vi "Write X.vi"(8 "error in (no error)":errorcluster, 10 "X":variant, 11 "AssertEqualValue in":refnum<class "AssertEqualValue.lvclass">) -> (0 "error out":errorcluster, 3 "AssertEqualValue out":refnum<class "AssertEqualValue.lvclass">)   [LabVIEW 2021, in "Bananas.lvlib" / "AssertEqualValue.lvclass"]
uses:
  AssertEqualValue.lvclass
  AssertEqualValue.lvclass/AssertEqualValue.ctl
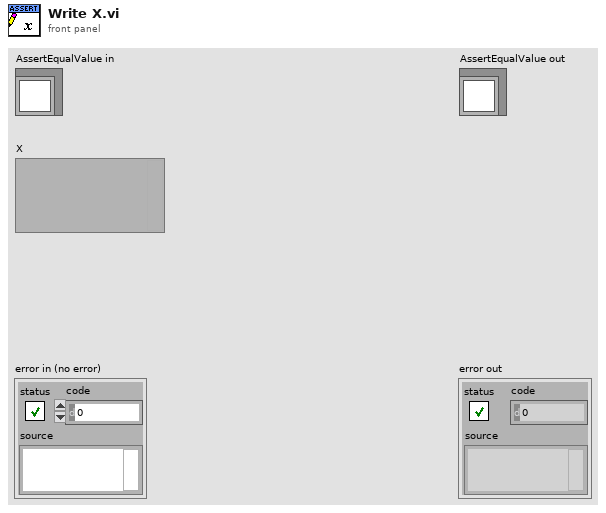
[diagram p1: front panel]
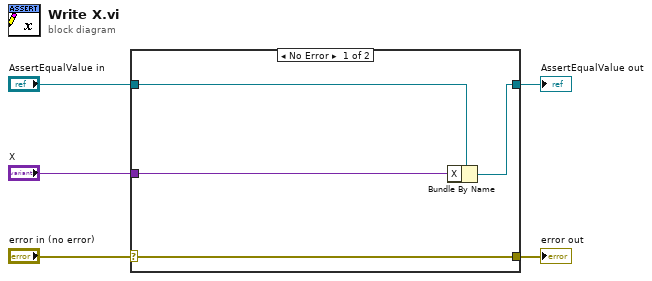
[diagram p0: block diagram]
diagram:
  n1 = case shown="No Error" "error in (no error)" {
    selector: "error in (no error)" -> [w9 w10]
    tunnel: [w9 w10] -> w4
    tunnel: [w7 w11] -> w2
    tunnel: "AssertEqualValue in" -> [w8 w11]
    tunnel: "X" -> [w6 _]
    frame No Error {
      n2 = Bundle By Name(cluster=w8, "X"=w6) -> (w7:refnum<class "AssertEqualValue.lvclass">)
    }
    frame Error {
    }
  }
  "error out" <- w4
  "AssertEqualValue out" <- w2
